vi "RESET ARM MOTORS.vi"(11 "ARM Climber range":T1) -> (1 "RESET SparkMAX":bool[](array[boolean]), 2 "RESET Phoenix":bool[](array[boolean]), 3 "RESET Phoenix 2":bool[](array[boolean]))   [LabVIEW 2020]
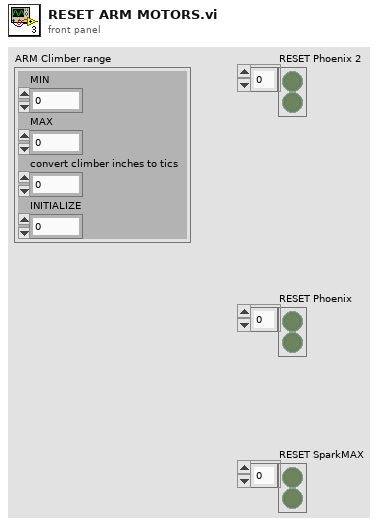
[diagram p1: front panel]
types:
  T1 = cluster{"MIN":dbl, "MAX":dbl, "convert climber inches to tics":dbl, "INITIALIZE":dbl}
  T2 = typedef "WPI_MotorControlDeviceRef.ctl" = cluster{"DeviceStatus":errorcluster, "Type":T3, "PWM":cluster{"PWM Channel":T4, "DeadBand":T5}, "CAN":cluster{"Device Number":u8, "SetOutput VI Ref":variant, "GetOutput VI Ref":variant, "Enable VI Ref":variant, "Disable VI Ref":variant, "Data":variant}, "Invert":bool, "DIO PWM":cluster{"PWM \"Enable\" Channel":T4, "DIOChannel":T6, "PWM Rate":dbl}}
  T3 = typedef "WPI_MotorControlType.ctl" = enum16{"PWM", "CAN", "DIO PWM"}
  T4 = typedef "FPGA_DIOPWMChannel.ctl" = enum8{"PWM 0", "PWM 1", "PWM 2", "PWM 3", "PWM 4", "PWM 5", "PWM 6", "PWM 7", "PWM 8", "PWM 9", "PWM MXP 0", "PWM MXP 1", "PWM MXP 2", "PWM MXP 3", "PWM MXP 4", "PWM MXP 5", "PWM MXP 6", "PWM MXP 7", "PWM MXP 8", "PWM MXP 9", "Invalid"}
  T5 = typedef "WPI_PWMDeadband.ctl" = cluster{"Name":string, "maxPositivePwm":i32, "minPositivePwm":i32, "centerPwm":i32, "maxNegativePwm":i32, "minNegativePwm":i32, "angularRange":u16}
  T6 = typedef "FPGA_DIOChannel.ctl" = enum8{"DIO 0", "DIO 1", "DIO 2", "DIO 3", "DIO 4", "DIO 5", "DIO 6", "DIO 7", "DIO 8", "DIO 9", "DIO MXP 0", "DIO MXP 1", "DIO MXP 2", "DIO MXP 3", "DIO MXP 4", "DIO MXP 5", "DIO MXP 6", "DIO MXP 7", "DIO MXP 8", "DIO MXP 9", "DIO MXP 10", "DIO MXP 11", "DIO MXP 12", "DIO MXP 13", "DIO MXP 14", "DIO MXP 15", "SPI Port CS1", "SPI Port CS2", "SPI Port CS3", "SPI Port MISO", "SPI Port MOSI", "Invalid"}
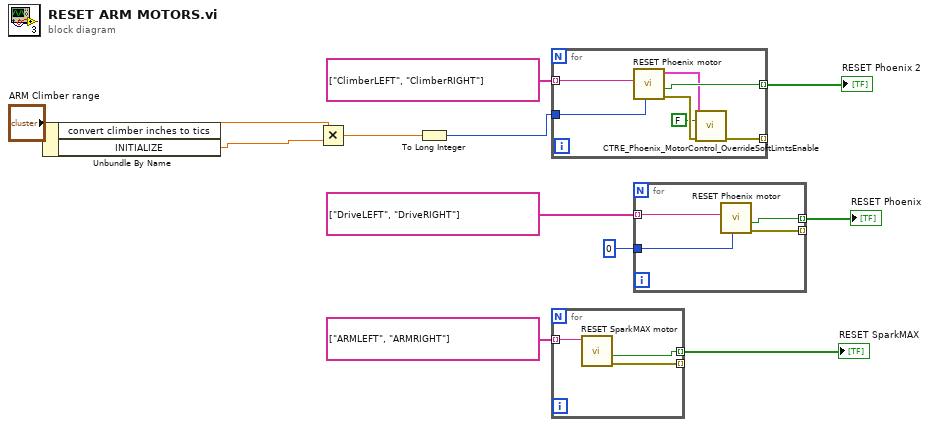
[diagram p0: block diagram]
diagram:
  n1 = Unbundle By Name("ARM Climber range") -> ("convert climber inches to tics"=w6:dbl, "INITIALIZE"=w12:dbl)
  n2 = Multiply(x=w6, y=w12) -> (x*y=w7:dbl)
  n3 = To Long Integer(number=w7) -> (32bit integer=w9:i32)
  n4 = for {
    tunnel: string[] ["ClimberLEFT", "ClimberRIGHT"] ("Phoenix motor refname") -> [w19] mode=indexing
    tunnel: [w18] -> w11 mode=indexing
    tunnel: w9 -> [w17]
    tunnel: [w15] -> _ mode=indexing
    n5 = call "RESET Phoenix motor.vi"("New Sensor Position"=w17, "Phoenix motor refname"=w19) -> ("error out"=w16:errorcluster, "RESET success?"=w18:bool, "PhoenixMotorControlDevRef"=w13:T2)  [unwired: 6 in, 1 out]
    n6 = call <vilib>:"CTRE_Phoenix_MotorControl_OverrideSoftLimtsEnable.vi"("PhoenixMotorControlDevRef"=w13, "Override Soft Limit Enable?"=FALSE, "error in (no error)"=w16) -> ("error out"=w15:errorcluster)  [unwired: 11 in, 1 out]
  }
  "RESET Phoenix 2" <- w11
  n7 = for {
    tunnel: string[] ["ARMLEFT", "ARMRIGHT"] ("Phoenix motor refname") -> [w22] mode=indexing
    tunnel: [w21] -> _ mode=indexing
    tunnel: [w20] -> w4 mode=indexing
    n8 = call "RESET SparkMAX motor.vi"("SparkMAX motor refname"=w22) -> ("error out"=w21:errorcluster, "RESET success?"=w20:bool)  [unwired: 7 in, 2 out]
  }
  "RESET SparkMAX" <- w4
  n9 = for {
    tunnel: string[] ["DriveLEFT", "DriveRIGHT"] ("Phoenix motor refname") -> [w26] mode=indexing
    tunnel: [w25] -> _ mode=indexing
    tunnel: [w24] -> w3 mode=indexing
    tunnel: 0 -> [w23]
    n10 = call "RESET Phoenix motor.vi"("New Sensor Position"=w23, "Phoenix motor refname"=w26) -> ("error out"=w25:errorcluster, "RESET success?"=w24:bool)  [unwired: 6 in, 2 out]
  }
  "RESET Phoenix" <- w3
